vi "Find Unique Indices_DBL.vi"(11 "Input Array":dbl[](array[numeric])) -> (2 "Unique indices":cluster{i32[]}[](array[cluster]), 3 "Unique values":dbl[](array[numeric]))   [LabVIEW 2015]
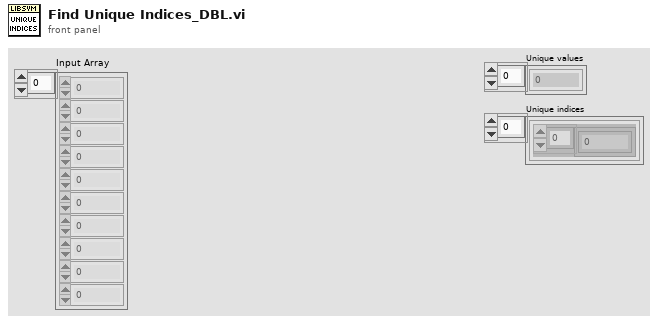
[diagram p1: front panel]
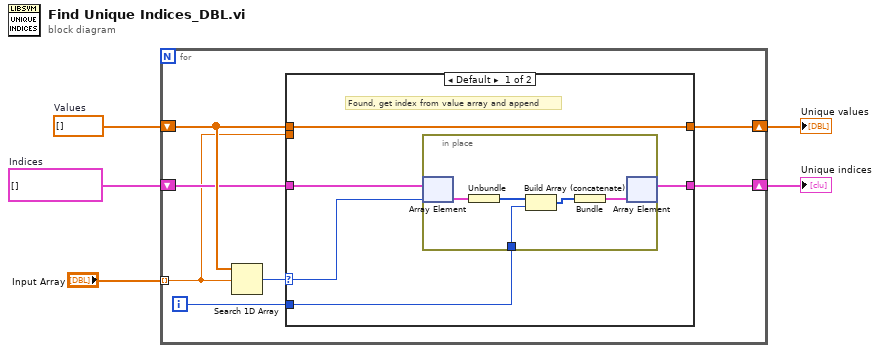
[diagram p0: block diagram]
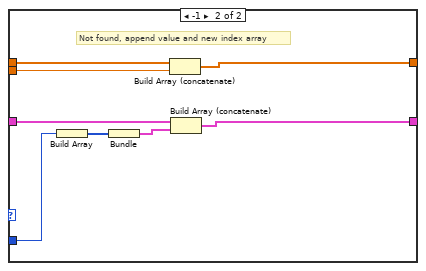
[diagram p2: hidden frame]
diagram:
  w3 = cluster{i32[]}[] []  # Indices
  w4 = dbl[] []  # Values
  n1 = for {
    shift-right: [w11] -> w2
    shift-left: w4 -> [w10]
    tunnel: "Input Array" -> [w6] mode=indexing
    shift-right: [w8] -> w1
    shift-left: w3 -> [w9]
    i -> [w7]
    n2 = Search 1D Array(1D array=w10, element=w6) -> (index of element=w12:i32)  [unwired: 1 in]
    n3 = case shown="Default" w12 {
      selector: w12 -> [w14 _]
      tunnel: [w17 w30] -> w11
      tunnel: w10 -> [w17 w29]
      tunnel: w9 -> [w16 w28]
      tunnel: [w15 w25] -> w8
      tunnel: w7 -> [w13 w24]
      tunnel: w6 -> [_ w23]
      frame Default {
        # "Found, get index from value array and append"
        n4 = in-place {
          in-place-border: w13 -> [w18]
          n5 = in-place-array #1(w16, w14) -> (w22:cluster{i32[]})
          n6 = Unbundle(w22) -> (w21:i32[])
          n7 = Build Array (concatenate)(w21, w18) -> (w20:i32[])
          n8 = Bundle(w20) -> (w19:cluster{i32[]})  [unwired: 1 in]
          n9 = in-place-array #1(w19) -> (w15:cluster{i32[]}[])  [unwired: 1 out]
        }
      }
      frame -1 {
        # "Not found, append value and new index array"
        n10 = Build Array(w24) -> (w27:i32[])
        n11 = Bundle(w27) -> (w26:cluster{i32[]})  [unwired: 1 in]
        n12 = Build Array (concatenate)(w29, w23) -> (w30:dbl[])
        n13 = Build Array (concatenate)(w28, w26) -> (w25:cluster{i32[]}[])
      }
    }
  }
  "Unique values" <- w2
  "Unique indices" <- w1
